vi "DB_Search Record.vi"() -> ()   [LabVIEW 2013, in "ConfigDBLib.lvlib"]
uses:
  ConfigDBLib.lvlib
panel:
  out "error out":errorcluster
  in  "error in (no error)":errorcluster
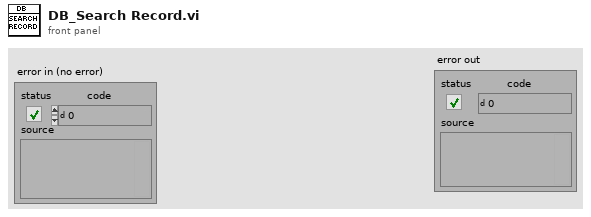
[diagram p1: front panel]
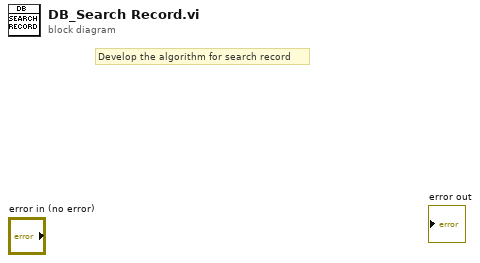
[diagram p0: block diagram]
diagram:
  # "Develop the algorithm for search record"
